vi "Pull_Data_from_Server.vi"(2 "Files to Pull":path[](array[path]), 3 "Relative Path":path) -> (0 "error out":errorcluster, 1 "Zip File String":string)   [LabVIEW 2011]
uses:
  Anemometry/Anemometry Sub Vis/Globals/Constants_global.vi
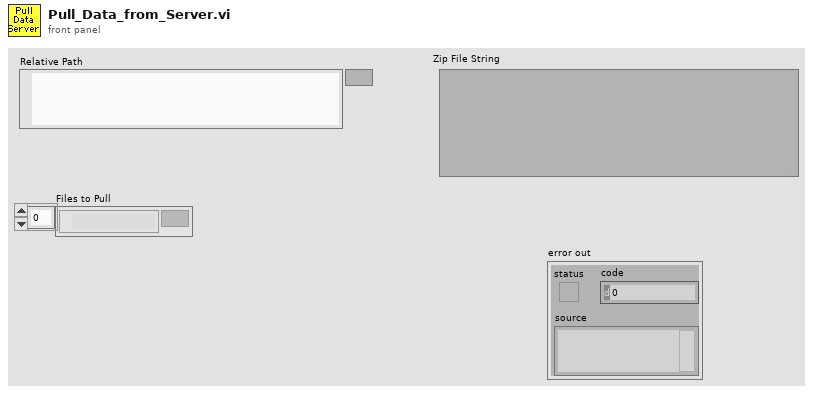
[diagram p1: front panel]
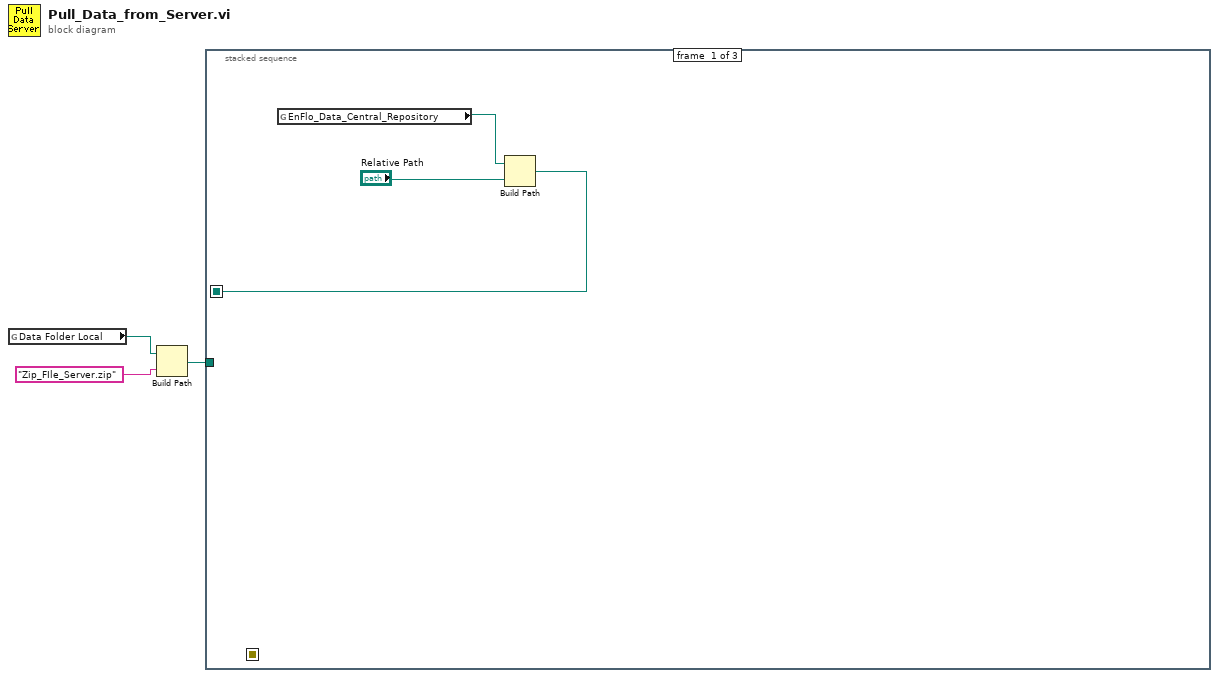
[diagram p0: block diagram]
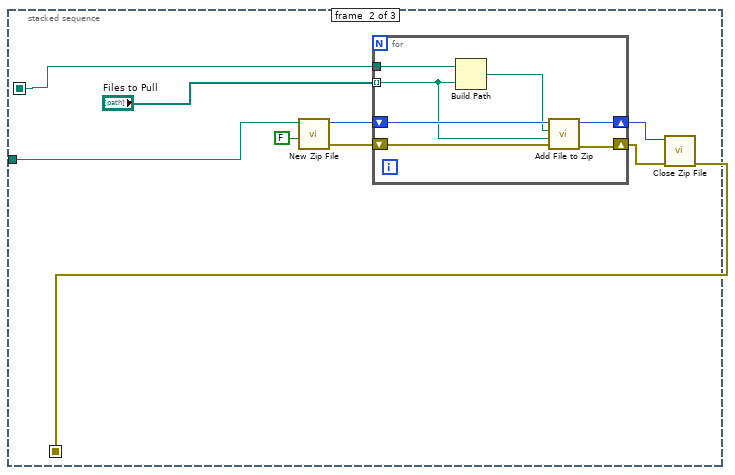
[diagram p2: hidden frame]
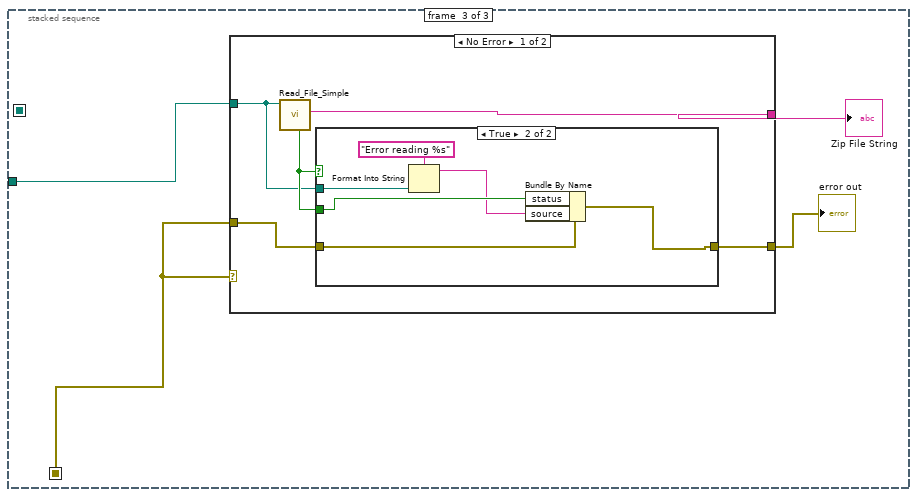
[diagram p3: hidden frame]
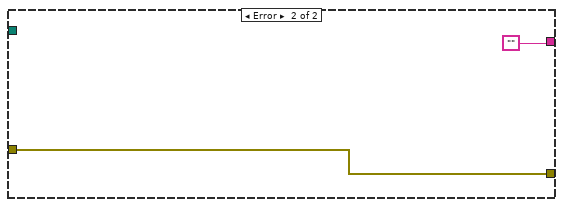
[diagram p5: hidden frame]
diagram:
  n1 = global read "Constants_global.vi" "Data Folder Local"() -> (w3:path)
  n2 = Build Path(base path=w3, name or relative path="Zip_FIle_Server.zip") -> (appended path=w1:path)
  n3 = stacked-sequence {
    seq-local: [w6 _ _] -> [_ w11 _]
    seq-local: [_ w7 _] -> [_ _ w24]
    tunnel: w1 -> [_ w10 w26]
    frame #0 {
      n4 = global read "Constants_global.vi" "EnFlo_Data_Central_Repository"() -> (w4:path)
      n5 = Build Path(base path=w4, name or relative path="Relative Path") -> (appended path=w6:path)
    }
    frame #1 {
      n6 = call <vilib>:"New Zip File.vi"("confirm overwrite? (F)"=FALSE, "target"=w10) -> ("error out"=w9:errorcluster, "zip file out"=w14:i64)  [unwired: 3 in, 1 out]
      n7 = for {
        shift-right: [w21] -> w13
        shift-left: w14 -> [w22]
        tunnel: w11 -> [w20]
        tunnel: "Files to Pull" -> [w18] mode=indexing
        shift-right: [w16] -> w8
        shift-left: w9 -> [w17]
        n8 = Build Path(base path=w20, name or relative path=w18) -> (appended path=w19:path)
        n9 = call <vilib>:"Add File to Zip.vi"("error in (no error)"=w17, "destination path in zip"=w18, "source file path"=w19, "zip file in"=w22) -> ("error out"=w16:errorcluster, "zip file out"=w21:i64)  [unwired: 6 in]
      }
      n10 = call <vilib>:"Close Zip File.vi"("error in (no error)"=w8, "zip file in"=w13) -> ("error out"=w7:errorcluster)  [unwired: 5 in]
    }
    frame #2 {
      n11 = case shown="No Error" w24 {
        tunnel: w26 -> [w28 _]
        tunnel: [w31 ""] -> w25
        tunnel: w24 -> [w30 w40]
        tunnel: [w27 w40] -> w23
        frame No Error {
          n12 = call "Read_File_Simple.vi"("Filename"=w28) -> ("Error?"=w29:bool, "string"=w31:string)  [unwired: 4 in, 4 out]
          n13 = case shown="True" w29 {
            tunnel: w30 -> [w32 w38]
            tunnel: w29 -> [_ w37]
            tunnel: w28 -> [_ w35]
            tunnel: [w32 w33] -> w27
            frame False {
            }
            frame True {
              n14 = Format Into String(format string="Error reading %s", w35) -> (resulting string=w34:string)  [unwired: 2 in, 1 out]
              n15 = Bundle By Name(cluster=w38, "status"=w37, "source"=w34) -> (w33:errorcluster)
            }
          }
        }
        frame Error {
        }
      }
      "Zip File String" <- w25
      "error out" <- w23
    }
  }
